vi "Get signal type.vi"(8 "error in (no error)":errorcluster, 11 "Generator in":refnum<class "Generador.lvclass">) -> (0 "error out":errorcluster, 2 "signal type":T1(ring), 3 "Generator out":refnum<class "Generador.lvclass">)   [LabVIEW 2020, in "FGen.lvlib" / "Generador.lvclass"]
uses:
  Generador.lvclass
  Generador.lvclass/Generador.ctl
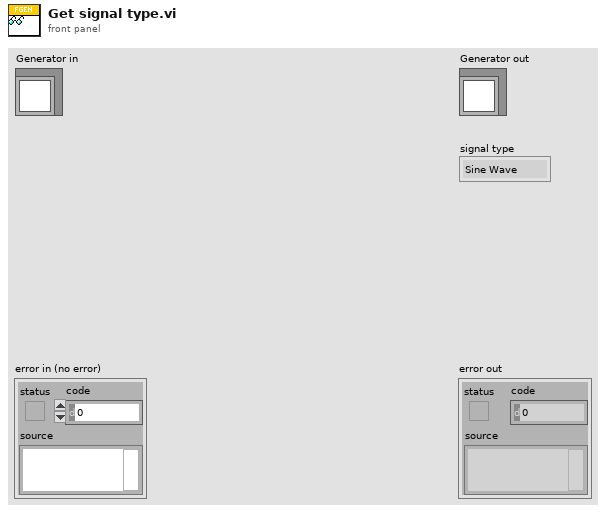
[diagram p1: front panel]
types:
  T1 = enum16{"Sine Wave", "Triangle Wave", "Square Wave", "Sawtooth Wave"}
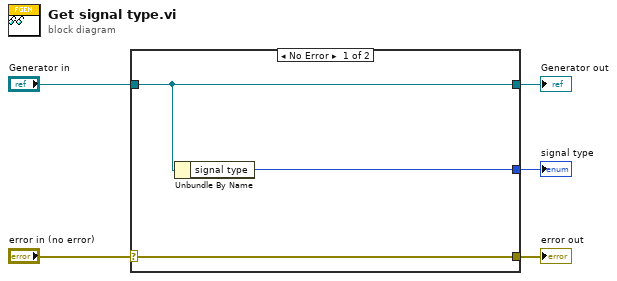
[diagram p0: block diagram]
diagram:
  n1 = case shown="No Error" "error in (no error)" {
    selector: "error in (no error)" -> [w8 w9]
    tunnel: [w8 w9] -> w4
    tunnel: [w7 w10] -> w2
    tunnel: "Generator in" -> [w7 w10]
    tunnel: [w6 _] -> w1
    frame No Error {
      n2 = Unbundle By Name(w7) -> ("signal type"=w6:T1)
    }
    frame Error {
    }
  }
  "error out" <- w4
  "Generator out" <- w2
  "signal type" <- w1
